vi "StopControl.vi"(8 "WindowButton":refnum<vi>, 9 "StopButton":refnum<vi>, 10 "Window mode notifier in":refnum<notifier>, 11 "Stop Notifier in":refnum<notifier>) -> ()   [LabVIEW 2015]
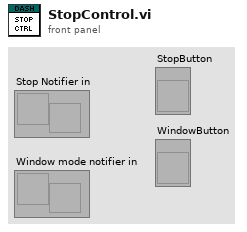
[diagram p1: front panel]
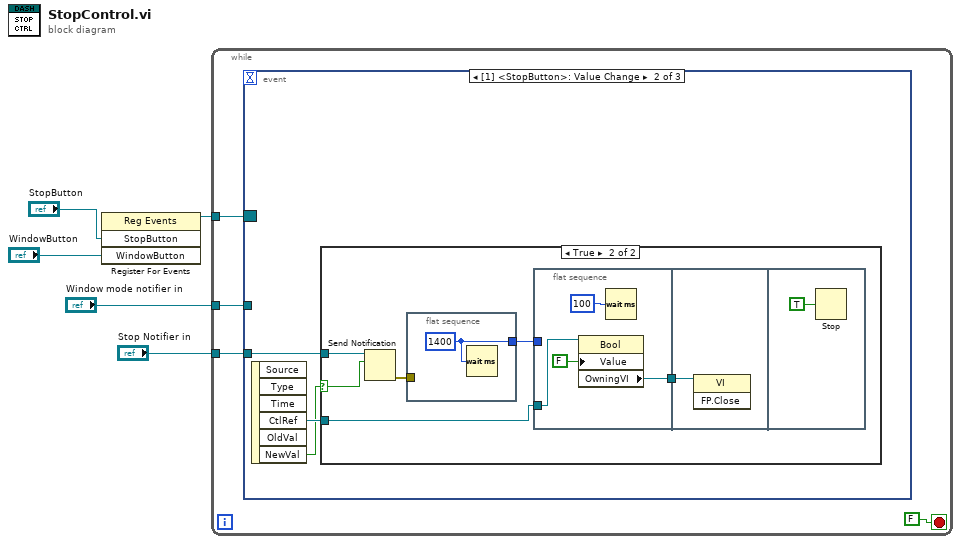
[diagram p0: block diagram]
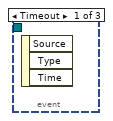
[diagram p2: hidden frame]
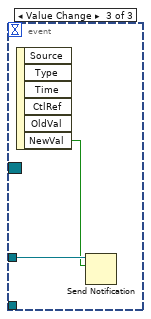
[diagram p4: hidden frame]
diagram:
  n1 = register-events("StopButton", "WindowButton") -> (reference out=w2:refnum<event-registration>)  [unwired: 2 in, 1 out]
  n2 = while {
    tunnel: "Window mode notifier in" -> [w8]
    tunnel: "Stop Notifier in" -> [w7]
    tunnel: w2 -> [w6]
    stop <- FALSE stop-if-true
    n3 = event shown="[1] <StopButton>: Value Change" {
      selector: w6 -> [_ _ _]
      dyn-events: _ -> [_ _ _]
      timeout: _ -> [_ _ _]
      tunnel: w8 -> [_ _ w27]
      tunnel: w7 -> [_ w12 _]
      event Timeout {
        n4 = event-data() -> ()  [unwired: 1 in, 3 out]
      }
      event Value Change {
        n5 = event-data() -> ("CtlRef"=w11:refnum<vi>, "NewVal"=w10:bool)  [unwired: 1 in, 4 out]
        n6 = case shown="True" w10 {
          selector: w10 -> [_ w13]
          tunnel: w12 -> [_ w17]
          tunnel: w11 -> [_ w14]
          frame False {
          }
          frame True {
            n7 = Send Notification(notification=w13, notifier=w17) -> (error out=w16:errorcluster)  [unwired: 1 in, 1 out]
            n8 = flat-sequence {
              tunnel: w16 -> [_]
              tunnel: [w19] -> w15
              frame #0 {
                w19 = u32 1400 ("milliseconds to wait")
                n9 = Wait (ms)(milliseconds to wait=w19) -> ()  [unwired: 1 out]
              }
            }
            n10 = flat-sequence {
              tunnel: w15 -> [_]
              tunnel: w14 -> [w22]
              tunnel: [w20] -> w18
              tunnel: w18 -> [w24]
              frame #0 {
                n11 = property class="Bool"(reference=w22, "Value"=FALSE) -> ("OwningVI"=w20:refnum<vi>)  [unwired: 1 in, 2 out]
                n12 = Wait (ms)(milliseconds to wait=u32 100) -> ()  [unwired: 1 out]
              }
              frame #1 {
                n13 = invoke class="VI" method="FP.Close"(reference=w24) -> ()  [unwired: 2 in, 3 out]
              }
              frame #2 {
                n14 = Stop(stop? (T)=TRUE) -> ()
              }
            }
          }
        }
      }
      event Value Change {
        n15 = event-data() -> ("NewVal"=w26:bool)  [unwired: 1 in, 5 out]
        n16 = Send Notification(notification=w26, notifier=w27) -> ()  [unwired: 1 in, 2 out]
      }
    }
  }
